vi "GetPanName.vi"(8 "error in (no error)":errorcluster caption="entrée d'erreur (pas d'erreur)", 10 "PanelIndex":i32[](array[numeric]), 11 "LoadedDev In":refnum<class "BaseDevice.lvclass">[](array[class])) -> (0 "error out":errorcluster caption="sortie d'erreur", 2 "PanelNames":string[](array[string]), 3 "LoadedDev Out":refnum<class "BaseDevice.lvclass">[](array[class]))   [LabVIEW 2019, in "BaseDevice.lvclass"]
uses:
  BaseDevice.lvclass
  BaseDevice.lvclass/BaseDevice.ctl
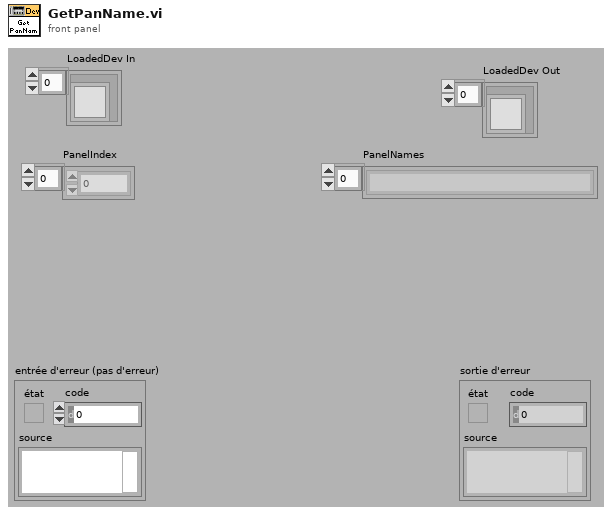
[diagram p1: front panel]
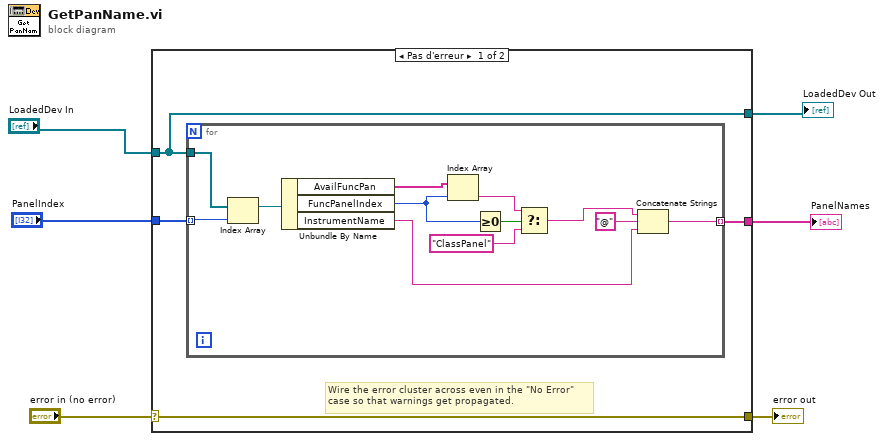
[diagram p0: block diagram]
diagram:
  n1 = case shown="Pas d'erreur" "error in (no error)" {
    selector: "error in (no error)" -> [w10 w24]
    tunnel: [w10 w24] -> w5
    tunnel: [w9 w23] -> w3
    tunnel: "LoadedDev In" -> [w9 w23]
    tunnel: [w8 _] -> w1
    tunnel: "PanelIndex" -> [w7 _]
    frame No Error {
      # "Wire the error cluster across even in the \"No Error\"\ncase so that warnings get propagated."
      n2 = for {
        tunnel: w9 -> [w22]
        tunnel: [w13] -> w8 mode=indexing
        tunnel: w7 -> [w11] mode=indexing
        n3 = Index Array(array=w22, index=w11) -> (element=w12:refnum<class "BaseDevice.lvclass">)
        n4 = Unbundle By Name(w12) -> ("AvailFuncPan"=w19:string[], "FuncPanelIndex"=w18:i32, "InstrumentName"=w14:string)
        n5 = Index Array(array=w19, index=w18) -> (element=w17:string)
        n6 = Greater Or Equal To 0?(x=w18) -> (x >= 0?=w21:bool)
        n7 = Select(t=w17, s=w21, f="ClassPanel") -> (s? t:f=w15:string)
        n8 = Concatenate Strings(w15, "@" ("chaîne"), w14) -> (w13:string)
      }
    }
    frame Error {
    }
  }
  "error out" <- w5
  "LoadedDev Out" <- w3
  "PanelNames" <- w1
